vi "Model - Get Elevator States.vi"(8 "error in (no error)":errorcluster, 11 "View Model":T2) -> (0 "error out":errorcluster, 1 "Next Elevator State":T1, 2 "Elevator State":T1, 3 "View Model":T2)   [LabVIEW 2017]
doc: "Get actual elevator states from DVR"
uses:
  Controls/View Model.ctl
  Error Handler/Controls/Error Model.ctl
  Error Handler/Controls/Error EventData.ctl
  Error Handler/Controls/Error Type.ctl
  Elevator Controller/Controls/Elevator Model.ctl
  Elevator Controller/Controls/Elevator Overhead.ctl
  Elevator Controller/Controls/Elevator States.ctl
  Elevator Controller/Controls/Elevator Location.ctl
  Elevator Controller/Controls/Elevator Command Event.ctl
  Elevator Controller/Controls/Elevator Commands.ctl
  Configuration/Controls/Configuration Model.ctl
  Configuration/Controls/Configuration Data.ctl
  Controls/Shared Model.ctl
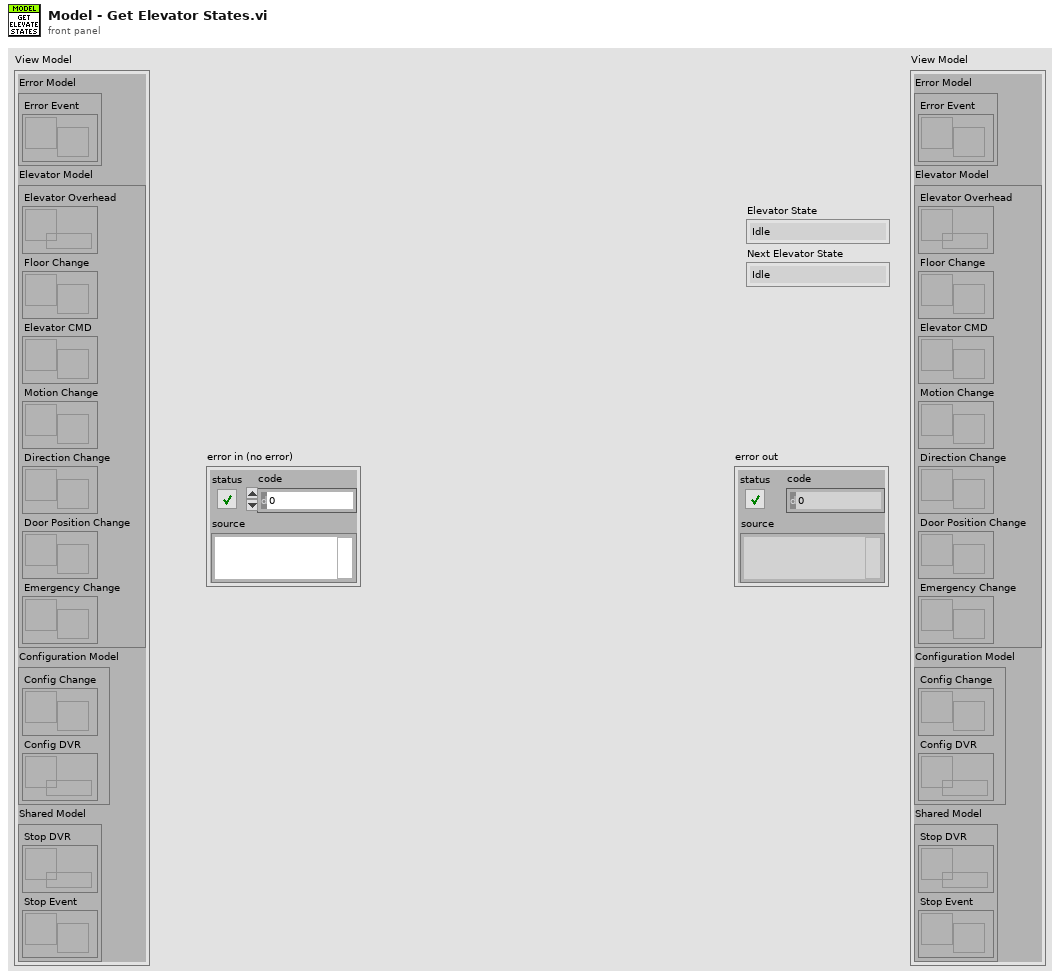
[diagram p1: front panel]
types:
  T1 = typedef "Elevator States.ctl" = enum16{"Idle", "Init", "Open Doors", "Close Doors", "Start Move", "Move", "Finish Move", "Analysis", "Emergency"}
  T2 = typedef "View Model.ctl" = cluster{"Error Model":T3, "Elevator Model":T4, "Configuration Model":T5, "Shared Model":T6}
  T3 = typedef "Error Model.ctl" = cluster{"Error Event":refnum<user-event>}
  T4 = typedef "Elevator Model.ctl" = cluster{"Elevator Overhead":refnum<data-value>, "Floor Change":refnum<user-event>, "Elevator CMD":refnum<user-event>, "Motion Change":refnum<user-event>, "Direction Change":refnum<user-event>, "Door Position Change":refnum<user-event>, "Emergency Change":refnum<user-event>}
  T5 = typedef "Configuration Model.ctl" = cluster{"Config Change":refnum<user-event>, "Config DVR":refnum<data-value>}
  T6 = typedef "Shared Model.ctl" = cluster{"Stop DVR":refnum<data-value>, "Stop Event":refnum<user-event>}
  T7 = typedef "Elevator Overhead.ctl" = cluster{"Elevator State":T1, "Next Elevator State":T1, "In Motion?":bool, "Direction":bool, "Door Movement":bool, "Door Position":bool, "Timer":dbl, "Elapsed Time":dbl}
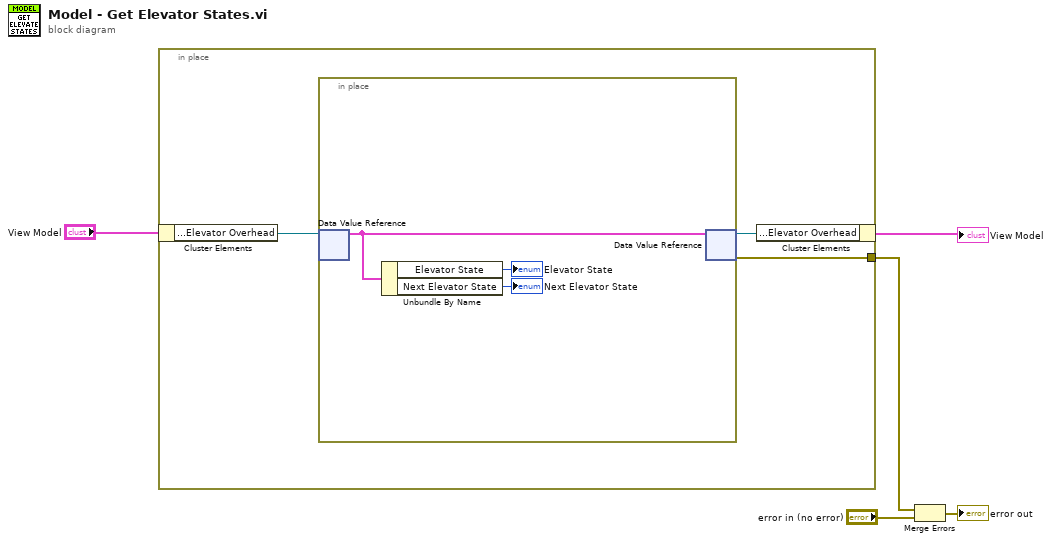
[diagram p0: block diagram]
diagram:
  n1 = in-place {
    in-place-border: [w7] -> w2
    n2 = in-place-cluster #1("View Model") -> ("Elevator Model.Elevator Overhead"=w6:refnum<data-value>)
    n3 = in-place {
      n4 = in-place-dvr #2(w6) -> (w11:T7)  [unwired: 1 out]
      n5 = Unbundle By Name(w11) -> ("Elevator State"=→"Elevator State":T1, "Next Elevator State"=→"Next Elevator State":T1)
      n6 = in-place-dvr #2(w11) -> (w8:refnum<data-value>, w7:errorcluster)
    }
    n7 = in-place-cluster #1("Elevator Model.Elevator Overhead"=w8) -> (→"View Model":T2)
  }
  n8 = Merge Errors(w2, "error in (no error)") -> (→"error out":errorcluster)
